vi "End1287.vi"(2 "Error In (No Error)":errorcluster, 3 "VISA Name In":refnum<visa-resource-name>="Solartron1287") -> (0 "error out":errorcluster, 1 "VISA resource name out":refnum<visa-resource-name>)   [LabVIEW 2018]
panel:
  # "Use for error handling; cannot be run without opening VISA session"
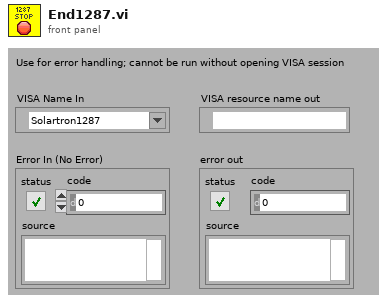
[diagram p1: front panel]
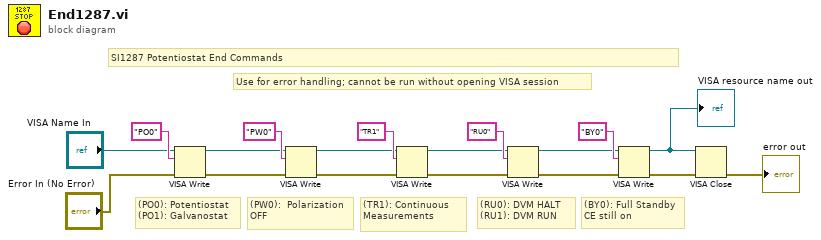
[diagram p0: block diagram]
diagram:
  # "Use for error handling; cannot be run without opening VISA session"
  # "(BY0): Full Standby\nCE still on"
  # "(RU0): DVM HALT\n(RU1): DVM RUN"
  # "(TR1): Continuous Measurements"
  # "(PW0):  Polarization OFF"
  # "(PO0): Potentiostat\n(PO1): Galvanostat"
  # "SI1287 Potentiostat End Commands"
  n1 = VISA Write(VISA resource name="VISA Name In", write buffer="PO0", error in (no error)="Error In (No Error)") -> (VISA resource name out=w13:refnum<visa-resource-name>, error out=w9:errorcluster)  [unwired: 1 out]
  n2 = VISA Write(VISA resource name=w13, write buffer="PW0", error in (no error)=w9) -> (VISA resource name out=w12:refnum<visa-resource-name>, error out=w8:errorcluster)  [unwired: 1 out]
  n3 = VISA Write(VISA resource name=w12, write buffer="TR1", error in (no error)=w8) -> (VISA resource name out=w11:refnum<visa-resource-name>, error out=w7:errorcluster)  [unwired: 1 out]
  n4 = VISA Write(VISA resource name=w11, write buffer="RU0", error in (no error)=w7) -> (VISA resource name out=w10:refnum<visa-resource-name>, error out=w6:errorcluster)  [unwired: 1 out]
  n5 = VISA Write(VISA resource name=w10, write buffer="BY0", error in (no error)=w6) -> (VISA resource name out=w2:refnum<visa-resource-name>, error out=w3:errorcluster)  [unwired: 1 out]
  "VISA resource name out" <- w2
  n6 = VISA Close(VISA resource name=w2, error in (no error)=w3) -> (error out=→"error out":errorcluster)
